vi "LED_Blue.vi"(9 "inten":dbl=2.0) -> ()   [LabVIEW 2012]
panel:
  in  "Blue":tag[](array[tag])
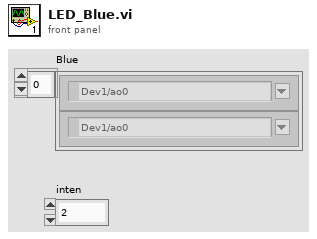
[diagram p1: front panel]
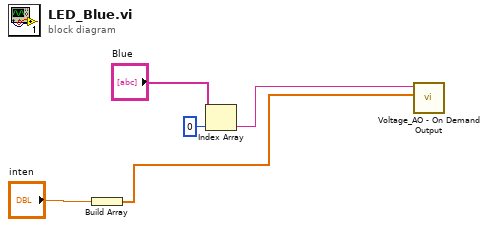
[diagram p0: block diagram]
diagram:
  n1 = Build Array("inten") -> (w1:dbl[])
  n2 = Index Array(array="Blue", index=0) -> (element=w3:tag)
  n3 = call "Voltage_AO - On Demand Output.vi"("Output Array"=w1, "Physical Channel(s)"=w3) -> ()  [unwired: 10 in]
